vi "GOOP_GetClassOverlayIcon.vi"(6 "DefaultIconName(BlueFull or InterfaceBlue)":string="BlueFull", 8 "error in (no error)":errorcluster, 10 "Item":T1, 11 "LVClassLibrary in":refnum<vi>) -> (0 "error out":errorcluster, 2 "IconName":string, 3 "LVClassLibrary out":refnum<vi>)   [LabVIEW 2020]
uses:
  <resource>/Framework/Providers/API/ItemRef.ctl
  <resource>/Framework/Providers/Open_GDS/ClassProviders/Common/LvClass_class/GDSLvClass_IconSettingsNames.ctl
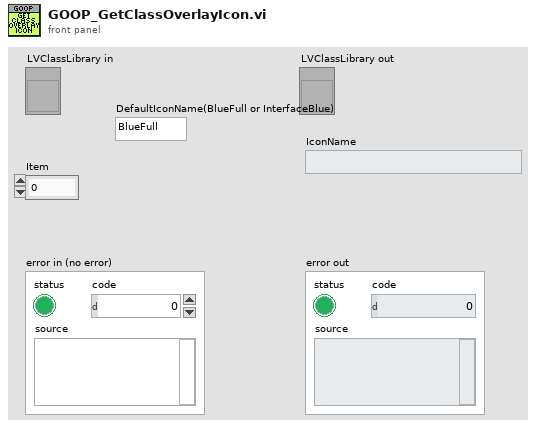
[diagram p1: front panel]
types:
  T1 = typedef "ItemRef.ctl" = u64
  T2 = typedef "GDSLvClass_IconSettingsNames.ctl" = enum16{"EndevoGOOP_ColorFrame", "EndevoGOOP_FrameThickness", "EndevoGOOP_ColorHeader", "EndevoGOOP_ColorTextHeader", "EndevoGOOP_ColorPublic", "EndevoGOOP_ColorProtected", "EndevoGOOP_ColorPrivate", "EndevoGOOP_ColorTextBody", "EndevoGOOP_ClassItemIcon", "EndevoGOOP_ClassBodyIcon"}
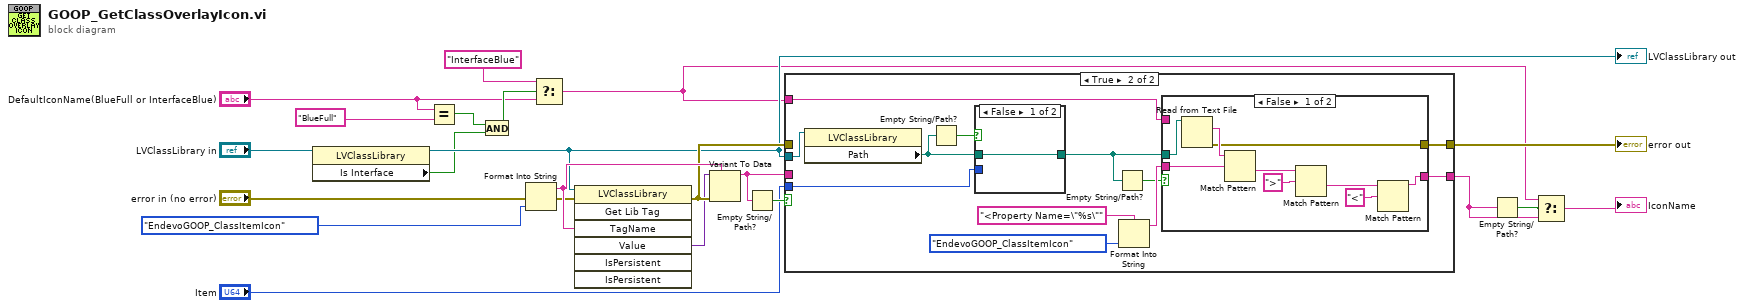
[diagram p0: block diagram]
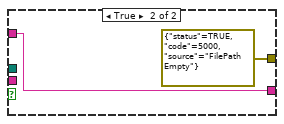
[diagram p3: hidden frame]
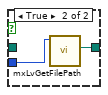
[diagram p4: hidden frame]
diagram:
  n1 = property class="LVClassLibrary"(reference="LVClassLibrary in") -> (reference out=w8:refnum<vi>, "Is Interface"=w7:bool)  [unwired: 1 in, 1 out]
  "LVClassLibrary out" <- w8
  n2 = Equal?(x="DefaultIconName(BlueFull or InterfaceBlue)", y="BlueFull" ("DefaultIconName(BlueFull)")) -> (x = y?=w5:bool)
  n3 = And(x=w5, y=w7) -> (x .and. y?=w4:bool)
  n4 = Format Into String(error in="error in (no error)", GDSLvClass_IconSettingsNames."EndevoGOOP_ClassItemIcon" ("Enum")) -> (resulting string=w21:string, error out=w18:errorcluster)  [unwired: 2 in]
  n5 = Select(t="InterfaceBlue" ("DefaultIconName(BlueFull)"), s=w4, f="DefaultIconName(BlueFull or InterfaceBlue)") -> (s? t:f=w2:string)
  n6 = invoke class="LVClassLibrary" method="Get Lib Tag"(reference=w8, error in=w18, "TagName"=w21) -> (error out=w20:errorcluster, "Value"=w16:variant)  [unwired: 4 in, 5 out]
  n7 = Variant To Data(error in=w20, type=w21, Variant=w16) -> (data=w22:string)  [unwired: 1 out]
  n8 = Empty String/Path?(string/path=w22) -> (empty?=w19:bool)
  n9 = case shown="True" w19 {
    tunnel: w8 -> [_ w36]
    tunnel: w20 -> [w23 _]
    tunnel: [w24 w32] -> w11
    tunnel: w22 -> [w24 _]
    tunnel: [w23 w31] -> w13
    tunnel: "Item" -> [_ w29]
    tunnel: w2 -> [_ w25]
    frame False {
    }
    frame True {
      n10 = property class="LVClassLibrary"(reference=w36) -> ("Path"=w28:path)  [unwired: 1 in, 2 out]
      n11 = Empty String/Path?(string/path=w28) -> (empty?=w30:bool)
      n12 = case shown="False" w30 {
        tunnel: w29 -> [_ w50]
        tunnel: [w48 w49] -> w27
        tunnel: w28 -> [w48 _]
        frame False {
        }
        frame True {
          n13 = call <resource>:"mxLvGetFilePath.vi"("Item"=w50) -> ("File Path"=w49:path)  [unwired: 8 in, 2 out]
        }
      }
      n14 = Empty String/Path?(string/path=w27) -> (empty?=w26:bool)
      n15 = Format Into String(format string="<Property Name=\"%s\"", GDSLvClass_IconSettingsNames."EndevoGOOP_ClassItemIcon" ("Enum")) -> (resulting string=w33:string)  [unwired: 2 in, 1 out]
      n16 = case shown="False" w26 {
        tunnel: w33 -> [w41 _]
        tunnel: [w39 w46] -> w32
        tunnel: [w38 errorcluster {"status"=TRUE, "code"=5000, "source"="FilePath Empty"} ("error out")] -> w31
        tunnel: w27 -> [w37 _]
        tunnel: w25 -> [_ w46]
        frame False {
          n17 = Read from Text File(file (use dialog)=w37) -> (text=w40:string, error out=w38:errorcluster)  [unwired: 3 in, 2 out]
          n18 = Match Pattern(string=w40, regular expression=w41) -> (after substring=w44:string)  [unwired: 1 in, 3 out]
          n19 = Match Pattern(string=w44, regular expression=">") -> (after substring=w45:string)  [unwired: 1 in, 3 out]
          n20 = Match Pattern(string=w45, regular expression="<") -> (before substring=w39:string)  [unwired: 1 in, 3 out]
        }
        frame True {
        }
      }
    }
  }
  "error out" <- w13
  n21 = Empty String/Path?(string/path=w11) -> (empty?=w12:bool)
  n22 = Select(t=w2, s=w12, f=w11) -> (s? t:f=→"IconName":string)
